vi "Configure Jitter Measurement.vi"   [LabVIEW 2015, in "Agilent 2000 3000 X-Series.lvlib"]
doc: "Jitter Measurement Polymorphic VI"
uses:
  <instrlib>/Agilent 2000 3000 X-Series/Agilent 2000 3000 X-Series.lvlib
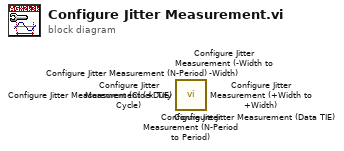
[diagram p0: block diagram]
diagram:
  n1 = call <instrlib>:"Configure Jitter Measurement (N-Period to Period).vi"() -> ()  [unwired: 10 in, 2 out]
  n2 = call <instrlib>:"Configure Jitter Measurement (-Width to -Width).vi"() -> ()  [unwired: 10 in, 2 out]
  n3 = call <instrlib>:"Configure Jitter Measurement (+Duty Cycle).vi"() -> ()  [unwired: 10 in, 2 out]
  n4 = call <instrlib>:"Configure Jitter Measurement (+Width to +Width).vi"() -> ()  [unwired: 10 in, 2 out]
  n5 = call <instrlib>:"Configure Jitter Measurement (N-Period).vi"() -> ()  [unwired: 10 in, 2 out]
  n6 = call <instrlib>:"Configure Jitter Measurement (Data TIE).vi"() -> ()  [unwired: 10 in, 2 out]
  n7 = call <instrlib>:"Configure Jitter Measurement (Clock TIE).vi"() -> ()  [unwired: 10 in, 2 out]
